vi "Convert Polygon to ROI(Rectangle).vi"(8 "error in (no error)":errorcluster, 11 "Rectangle Points":T1[](array[typedef])=[{"X"=194.0, "Y"=132.0}, {"X"=460.0, "Y"=60.0}, {"X"=493.0, "Y"=182.0}, {"X"=227.0, "Y"=254.0}, {"X"=194.0, "Y"=132.0}] {"Y" format="%.2f"; "X" format="%.2f"}) -> (0 "error out":errorcluster, 3 "ROI Descriptor":T2 {"Contours"."Type" items=["No Selection", "Point", "Line", "Rectangle", "Oval", "Polygon", "Freehand Region", "Annulus", "Unused2", "Unused3", "Broken Line", "Freehand Line", "Rotated Rectangle"]})   [LabVIEW 2015]
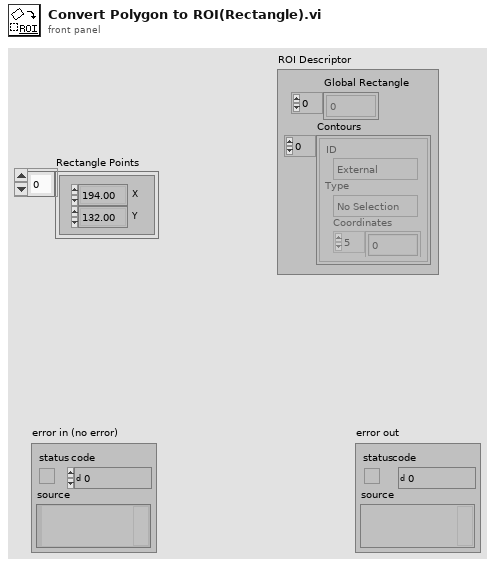
[diagram p1: front panel]
types:
  T1 = typedef "IMAQ Point" = cluster{"X":sgl, "Y":sgl}
  T2 = typedef "ROI Descriptor" = cluster{"Global Rectangle":i32[], "Contours":cluster{"ID":enum32{"External", "Internal"}, "Type":u32, "Coordinates":i32[]}[]}
  T3 = cluster{"ID":enum32{"External", "Internal"}, "Type":u32, dbl[]}
  T4 = cluster{"ID":enum32{"External", "Internal"}, "Type":u32, dbl[]}[]
  T5 = cluster{i32[], cluster{"ID":enum32{"External", "Internal"}, "Type":u32, dbl[]}[]}
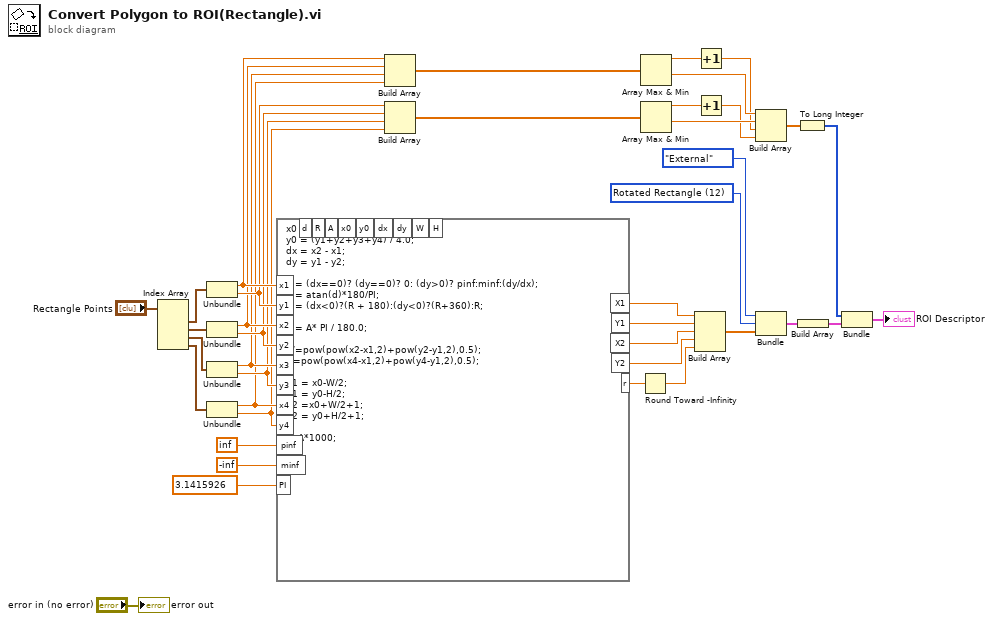
[diagram p0: block diagram]
diagram:
  w25 = u32 12 items=["No Selection", "Point", "Line", "Rectangle", "Oval", "Polygon", "Freehand Region", "Annulus", "Unused2", "Unused3", "Broken Line", "Freehand Line", "Rotated Rectangle"] ("Type")
  n1 = Index Array(array="Rectangle Points") -> (element #1=w38:T1, element #2=w37:T1, element #3=w36:T1, element #4=w35:T1)  [unwired: 4 in]
  n2 = Unbundle(w38) -> ("X"=w17:sgl, "Y"=w16:sgl)
  n3 = Unbundle(w37) -> ("X"=w15:sgl, "Y"=w14:sgl)
  n4 = Unbundle(w36) -> ("X"=w13:sgl, "Y"=w12:sgl)
  n5 = Unbundle(w35) -> ("X"=w11:sgl, "Y"=w10:sgl)
  n6 = formula code="x0 = (x1+x2+x3+x4) / 4.0;\ny0 = (y1+y2+y3+y4) / 4.0;\ndx = x2 - x1;\ndy = y1 - y2;\n\nd = (dx==0)? (dy==0)? 0: (dy>0)? pinf:minf:(dy/dx);\nR = atan(d)*180/PI;\nA = (dx<0)?(R + 180):(dy<0)?(R+360):R;\n\nR = A* PI / 180.0;\n\nW=pow(pow(x2-x1,2)+pow(y2-y1,2),0.5);\nH=pow(pow(x4-x1,2)+pow(y4-y1,2),0.5);\n\nX1 = x0-W/2;\nY1 = y0-H/2;\nX2 =x0+W/2+1;\nY2 = y0+H/2+1;\n\nr=A*1000;"("x1"=w17, "y1"=w16, "x2"=w15, "y2"=w14, "x3"=w13, "y3"=w12, "x4"=w11, "y4"=w10, "pinf"=inf, "minf"=-inf, "PI"=3.1415926 ("input variable")) -> ("X1"=w7:dbl, "Y1"=w6:dbl, "X2"=w5:dbl, "Y2"=w4:dbl, "r"=w3:dbl)  [unwired: 9 out]
  n7 = Build Array(w17, w15, w13, w11) -> (w34:sgl[])
  n8 = Build Array(w16, w14, w12, w10) -> (w33:sgl[])
  n9 = Round Toward -Infinity(1:w3) -> (0:w23:dbl)
  n10 = Array Max & Min(array=w34) -> (max value=w21:sgl, min value=w32:sgl)  [unwired: 2 out]
  n11 = Array Max & Min(array=w33) -> (max value=w19:sgl, min value=w31:sgl)  [unwired: 2 out]
  n12 = Build Array(w7, w6, w5, w4, w23) -> (w22:dbl[])
  n13 = Increment(x=w21) -> (x+1=w20:sgl)
  n14 = Increment(x=w19) -> (x+1=w18:sgl)
  n15 = Build Array(w32, w31, w20, w18) -> (w30:sgl[])
  n16 = Bundle("ID"=enum32{"External", "Internal"}."External", "Type"=w25, w22) -> (w27:T3)  [unwired: 1 in]
  n17 = To Long Integer(number=w30) -> (32bit integer=w24:i32[])
  n18 = Build Array(w27) -> (w28:T4)
  n19 = Bundle(w24, w28) -> (→"ROI Descriptor":T5)  [unwired: 1 in]
  "error out" <- "error in (no error)"
